vi "Initialize.vi"(8 "error in (no error)":errorcluster, 9 "thread settings":T1, 10 "transfer group configurations":T2[](array[typedef]) {"transfers"."channels"."string offset" format="%d bytes"}, 11 "PXImc Transceiver in":refnum<class "PXImc Transceiver.lvclass">) -> (0 "error out":errorcluster, 3 "PXImc Transceiver out":refnum<class "PXImc Transceiver.lvclass">)   [LabVIEW 2017, in "PXImc.lvlib" / "PXImc Transceiver.lvclass"]
uses:
  PXImc Transceiver.lvclass
  DSF Core.lvlibp/Typedefs/DSF Engine Transfer Group Configuration.ctl
  DSF Core.lvlibp/Typedefs/DSF Direction.ctl
  DSF Core.lvlibp/Typedefs/DSF Timing Info.ctl
  DSF Core.lvlibp/Typedefs/DSF Settings Info.ctl
  DSF Core.lvlibp/Typedefs/DSF Engine Transfer Configuration.ctl
  DSF Core.lvlibp/Typedefs/DSF Byte Order.ctl
  DSF Core.lvlibp/Typedefs/DSF Engine Channel Configuration.ctl
  DSF Core.lvlibp/Typedefs/DSF Data Type.ctl
  DSF Core.lvlibp/Typedefs/DSF Timeout Behavior.ctl
  DSF Core.lvlibp
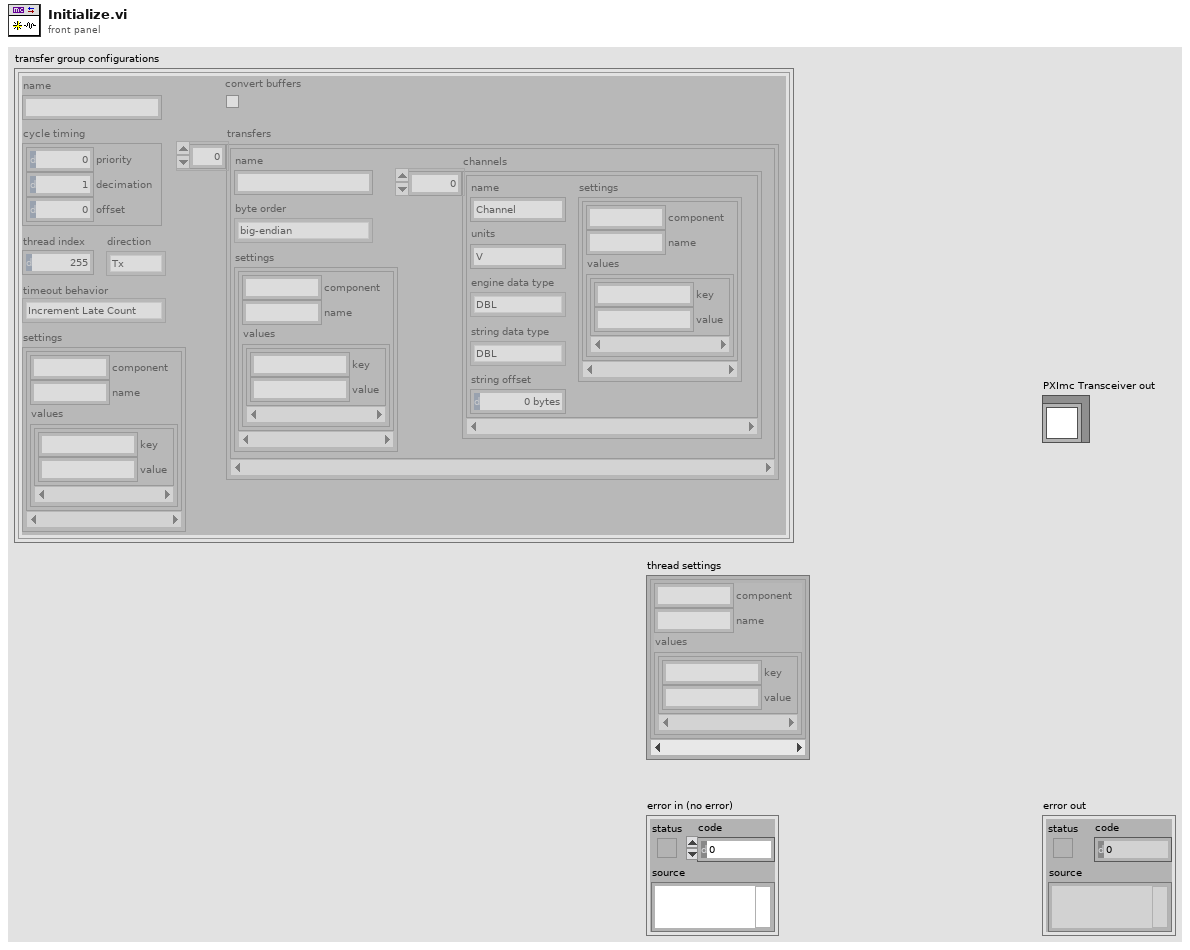
[diagram p1: front panel]
types:
  T1 = typedef "DSF Core.lvlibp/DSF Settings Info.ctl" = cluster{"component":string, "name":string, "values":cluster{"key":string, "value":string}[]}[]
  T2 = typedef "DSF Core.lvlibp/DSF Engine Transfer Group Configuration.ctl" = cluster{"name":string, "direction":T3, "cycle timing":T4, "thread index":u8, "settings":T1, "transfers":T5[], "timeout behavior":T9, "convert buffers":bool}
  T3 = typedef "DSF Core.lvlibp/DSF Direction.ctl" = enum8{"Tx", "Rx"}
  T4 = typedef "DSF Core.lvlibp/DSF Timing Info.ctl" = cluster{"priority":u64, "decimation":u64, "offset":u64}
  T5 = typedef "DSF Core.lvlibp/DSF Engine Transfer Configuration.ctl" = cluster{"name":string, "byte order":T6, "settings":T1, "channels":T7[]}
  T6 = typedef "DSF Core.lvlibp/DSF Byte Order.ctl" = enum8{"big-endian", "little-endian"}
  T7 = typedef "DSF Core.lvlibp/DSF Engine Channel Configuration.ctl" = cluster{"string offset":u64, "name":string, "units":string, "engine data type":T8, "string data type":T8, "settings":T1}
  T8 = typedef "DSF Core.lvlibp/DSF Data Type.ctl" = enum8{"Bool", "SGL", "DBL", "I8", "I16", "I32", "I64", "U8", "U16", "U32", "U64"}
  T9 = typedef "DSF Core.lvlibp/DSF Timeout Behavior.ctl" = enum8{"Increment Late Count", "Throw Error"}
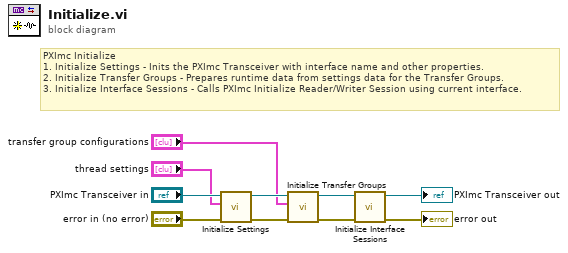
[diagram p0: block diagram]
diagram:
  # "PXImc Initialize\n1. Initialize Settings - Inits the PXImc Transceiver with interface name and other properties.\n2. Initialize Transfer Groups - Prepares runtime data from settings data for the Transfer Groups.\n3. Initialize Interface Sessions - Calls PXImc Initialize Reader/Writer Session using current interface."
  n1 = call "Initialize Settings.vi"("error in (no error)"="error in (no error)", "settings"="thread settings", "PXImc Transceiver in"="PXImc Transceiver in") -> ("error out"=w3:errorcluster, "PXImc Transceiver out"=w8:refnum<class "PXImc Transceiver.lvclass">)  [unwired: 7 in]
  n2 = call "Initialize Transfer Groups.vi"("error in (no error)"=w3, "Transfer Groups configurations"="transfer group configurations", "PXImc Transceiver in"=w8) -> ("error out"=w2:errorcluster, "PXImc Transceiver out"=w1:refnum<class "PXImc Transceiver.lvclass">)  [unwired: 7 in]
  n3 = call "Initialize Interface Sessions.vi"("error in (no error)"=w2, "PXImc Transceiver in"=w1) -> ("error out"=→"error out":errorcluster, "PXImc Transceiver out"=→"PXImc Transceiver out":refnum<class "PXImc Transceiver.lvclass">)  [unwired: 8 in]
